vi "Test.vi"() -> ()   [LabVIEW 2019]
panel:
  out "Boolean":bool
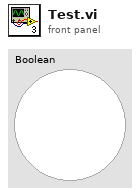
[diagram p1: front panel]
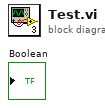
[diagram p0: block diagram]
diagram:
